vi "SysDef.Node.Pointer.Get.vi"(8 "error in (no error)":errorcluster, 11 "nodeID":u64) -> (0 "error out":errorcluster, 2 "Node Pointer":T1, 3 "nodeID out":u64, 4 "Found?":bool)   [LabVIEW 2016, in "Advanced System Definition.lvlib"]
uses:
  Advanced System Definition.lvlib
  <vilib>/NI Veristand/Custom Device API/Custom Device Pointer.ctl
  NationalInstruments.VeriStand.SystemStorage
  NationalInstruments.VeriStand.SystemDefinitionAPI
  <vilib>/NI VeriStand/Custom Device API/Custom Device API.lvlib
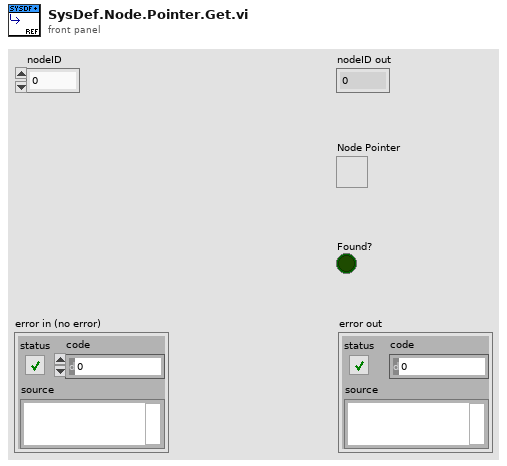
[diagram p1: front panel]
types:
  T1 = typedef "Custom Device API.lvlib/Custom Device Pointer.ctl" = refnum<k24>
  T2 = typedef "Custom Device API.lvlib/Custom Device Item Ref.ctl" = u64
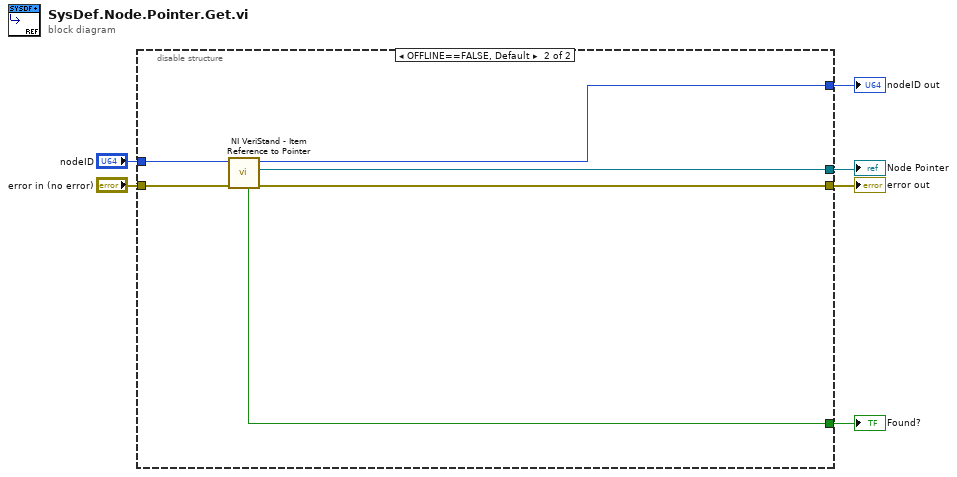
[diagram p0: block diagram]
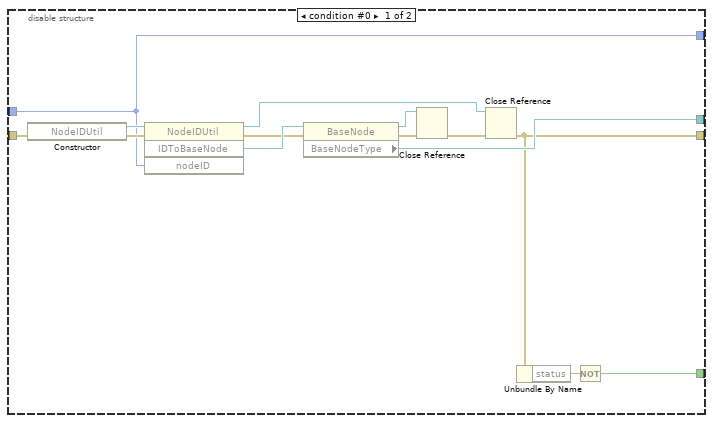
[diagram p2: hidden frame]
diagram:
  n1 = disable-structure shown="OFFLINE==FALSE, Default" {
    disable-tunnel: "error in (no error)" -> [w17 w22]
    disable-tunnel: "nodeID" -> [w14 w26]
    disable-tunnel: [w9 w24] -> w4
    disable-tunnel: [w7 w25] -> w3
    disable-tunnel: [w14 w23] -> w2
    disable-tunnel: [w10 w21] -> w1
    frame condition #0 {
      n2 = constructor class="NodeIDUtil"(error in=w17) -> (reference out=w20:refnum<k24>, error out=w19:errorcluster)  [unwired: 2 in, 1 out]
      n3 = invoke class="NodeIDUtil" method="IDToBaseNode"(reference=w20, error in=w19, "nodeID"=w14) -> (reference out=w11:refnum<k24>, error out=w13:errorcluster, "IDToBaseNode"=w18:refnum<k24>)  [unwired: 1 in, 1 out]
      n4 = property class="BaseNode"(reference=w18, error in=w13) -> (reference out=w16:refnum<k24>, error out=w15:errorcluster, "BaseNodeType"=w10:refnum<k24>)
      n5 = Close Reference(reference=w16, error in (no error)=w15) -> (error out=w12:errorcluster)
      n6 = Close Reference(reference=w11, error in (no error)=w12) -> (error out=w9:errorcluster)
      n7 = Unbundle By Name(w9) -> ("status"=w8:bool)
      n8 = Not(x=w8) -> (.not. x?=w7:bool)
    }
    frame condition #1 (active) {
      n9 = call <vilib>:"NI VeriStand - Item Reference to Pointer.vi"("error in (no error)"=w22, "Item Ref in"=w26) -> ("error out"=w24:errorcluster, "Node Pointer"=w21:T1, "Item Ref out"=w23:T2, "Found"=w25:bool)  [unwired: 6 in]
    }
  }
  "nodeID out" <- w2
  "error out" <- w4
  "Found?" <- w3
  "Node Pointer" <- w1
